vi "Flatten To MessagePack.vi"(8 "error in (no error)":errorcluster, 11 "Data":variant) -> (0 "error out":errorcluster, 3 "MsgPack Data":string)   [LabVIEW 2015, in "MsgPackSerializer.lvclass"]
uses:
  MsgPackSerializer.lvclass
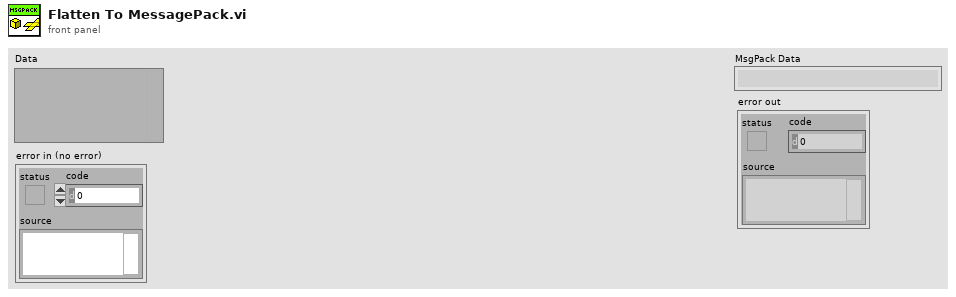
[diagram p1: front panel]
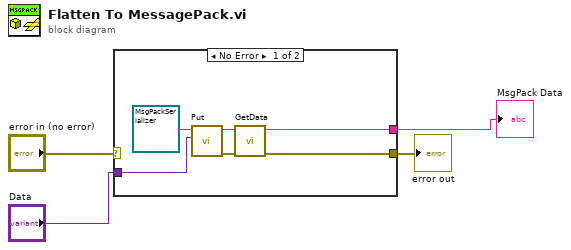
[diagram p0: block diagram]
diagram:
  n1 = case shown="No Error" "error in (no error)" {
    selector: "error in (no error)" -> [_ w11]
    tunnel: "Data" -> [w9 _]
    tunnel: [w6 w11] -> w3
    tunnel: [w5 _] -> w1
    frame No Error {
      n2 = call "Put.vi"("Data"=w9, "MsgPackSerializer in"=refnum<class "MsgPackSerializer.lvclass"> refnum) -> ("error out"=w8:errorcluster, "MsgPackSerializer out"=w7:refnum<class "MsgPackSerializer.lvclass">)  [unwired: 8 in]
      n3 = call "GetData.vi"("error in (no error)"=w8, "MsgPackSerializer in"=w7) -> ("error out"=w6:errorcluster, "Data"=w5:string)  [unwired: 8 in]
    }
    frame Error {
    }
  }
  "error out" <- w3
  "MsgPack Data" <- w1
